vi "DynamixelReadIDs.vi"() -> ()   [LabVIEW 2013]
uses:
  <instrlib>/Dynamixel Motor/Dynamixel Motor.lvlib
panel:
  out "Motors IDs Found":u8[](array[numeric])
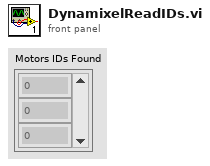
[diagram p1: front panel]
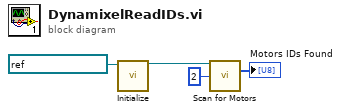
[diagram p0: block diagram]
diagram:
  n1 = call <instrlib>:"Initialize.vi"("VISA resource name"=refnum<visa-resource-name> "ASRL3::INSTR") -> ("VISA resource name out"=w3:refnum<visa-resource-name>)  [unwired: 9 in, 1 out]
  n2 = call <instrlib>:"Scan for Motors.vi"("VISA resource name"=w3, "Ending ID (253)"=u8 2) -> ("Motors IDs Found"=→"Motors IDs Found":u8[])  [unwired: 11 in, 2 out]
